vi "Test Driver.vi"() -> ()   [LabVIEW 2017]
uses:
  Controls/Test Driver States.ctl
  LabVIEW Library/Controls/Acquisition Modes.ctl
  LabVIEW Library/Controls/Acquisition Commands.ctl
  <vilib>/vision/Image Controls.llb/IMAQ Image.ctl
  builds/BonTechDetector.lvlibp
  LabVIEW Library/BonTechDetector.lvlib
  <vilib>/vision/NI_Vision_Development_Module.lvlib
panel:
  in  "byte order (0:big-endian, network order)":T1(ring)
  in  "Save Image":bool
  in  "Save File to":path
  out "SendCapCommand Status":i32 format="%.0x"
  in  "Acquisition Mode":T2(ring)
  in  "Stop Continuous Acquisition":bool
  in  "Start Continuous  Acquisition":bool
  in  "Acquisition Commands (nMode)":u16(ring) items=["ACQ_INIT"=0, "DARK_MODE"=1, "BRIGHT_MODE"=2, "SOFTTRIGGER_MODE"=258, "SOFTTRIGGER_INSTANT_MODE"=259]
  out "Continous Acq function Status":i32 format="%.0x"
  out "nHeight out":u32
  out "nWidth out":u32
  in  "Error in (no error)":errorcluster
  in  "Disconnect":bool
  in  "Capture Image":bool
  in  "Configure":bool
  in  "Connect":bool
  out "Capture Status":i32 format="%.0x"
  out "Image":T3(plugin-control)
  in  "CalRefPath":string="C:\\\\BSD\\\\192.168.3.240\\\\Reference"
  in  "ConfigDir":string="C:\\\\BSD\\\\192.168.3.240\\\\Config"
  out "lpszSerialNum out":string
  out "Acq Mode Set Status":i32 format="%.0x"
  out "Error out":errorcluster
  out "Disconnect Status":i32 format="%.0x"
  out "Connect Status":i32 format="%.0x"
  in  "nSensorIP":string="192.168.3.240"
  in  "nHostIP":string="192.168.3.5"
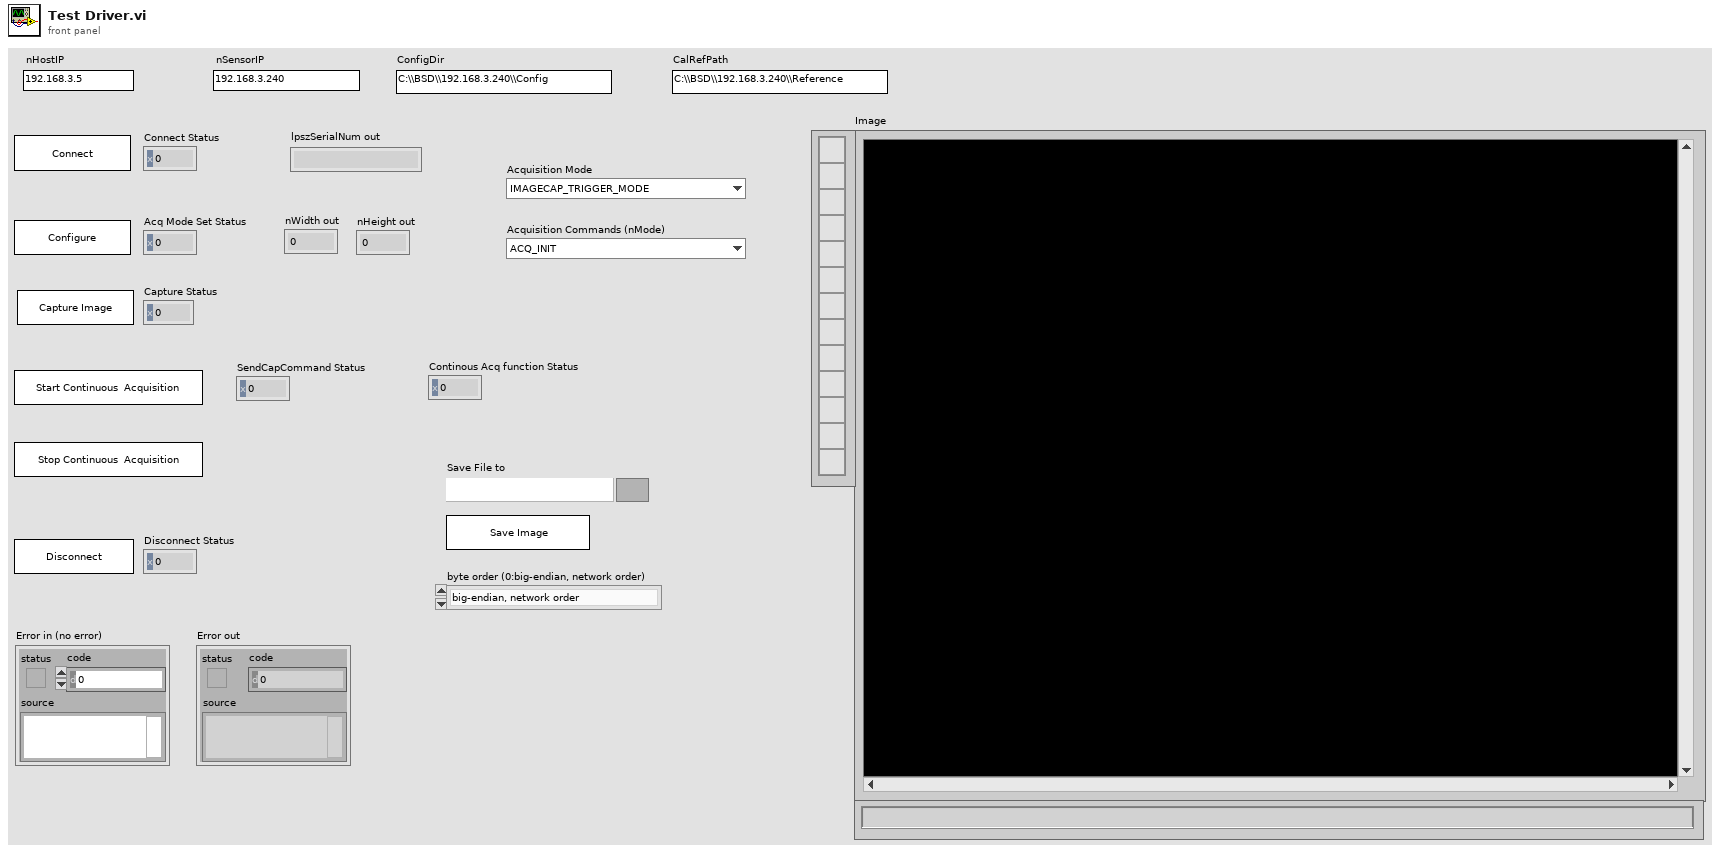
[diagram p1: front panel]
types:
  T1 = enum16{"big-endian, network order", "native, host order", "little-endian"}
  T2 = enum16{"IMAGECAP_TRIGGER_MODE", "IMAGECAP_AED_MODE", "IMAGECAP_SOFTTRIGGER_MODE", "IMAGECAP_AVG_COUNT_MODE", "IMAGECAP_AVG_AED_MODE", "IMAGECAP_CONTINUOUS_MODE", "IMAGECAP_CONTINUOUS_BINNING_MODE", "IMAGECAP_VIEWER_MODE"}
  T3 = typedef "IMAQ Image.ctl" = refnum<image>
  T4 = typedef "BonTechDetector.lvlib/Acquisition Modes.ctl" = enum32{"IMAGECAP_TRIGGER_MODE", "IMAGECAP_AED_MODE", "IMAGECAP_SOFTTRIGGER_MODE", "IMAGECAP_AVG_COUNT_MODE", "IMAGECAP_AVG_AED_MODE", "IMAGECAP_CONTINUOUS_MODE", "IMAGECAP_VIEWER_MODE", "IMAGECAP_CONTINUOUS_BINNING_MODE"}
  T5 = typedef "BonTechDetector.lvlib/Acquisition Commands.ctl" = u32
  T6 = cluster{"nHostIP String":string, "nSensorIP String":string, "ConfigDir":string, "CalRefPath":string, "nMode":T4, "nAcqCommand":T5, "pImage":u16[], "ImageRef":T3, "nWidth":u32, "nHeight":u32, "nHostIP":u32, "nSensorIP":u32, "imgCapQ":refnum<queue>}
  T7 = typedef "Test Driver States.ctl" = enum16{"Poll", "Init", "Connect", "Configure", "Capture Image", "Save Image", "Disconnect", "Error", "Exit"}
  T8 = typedef "Image Type" = u32
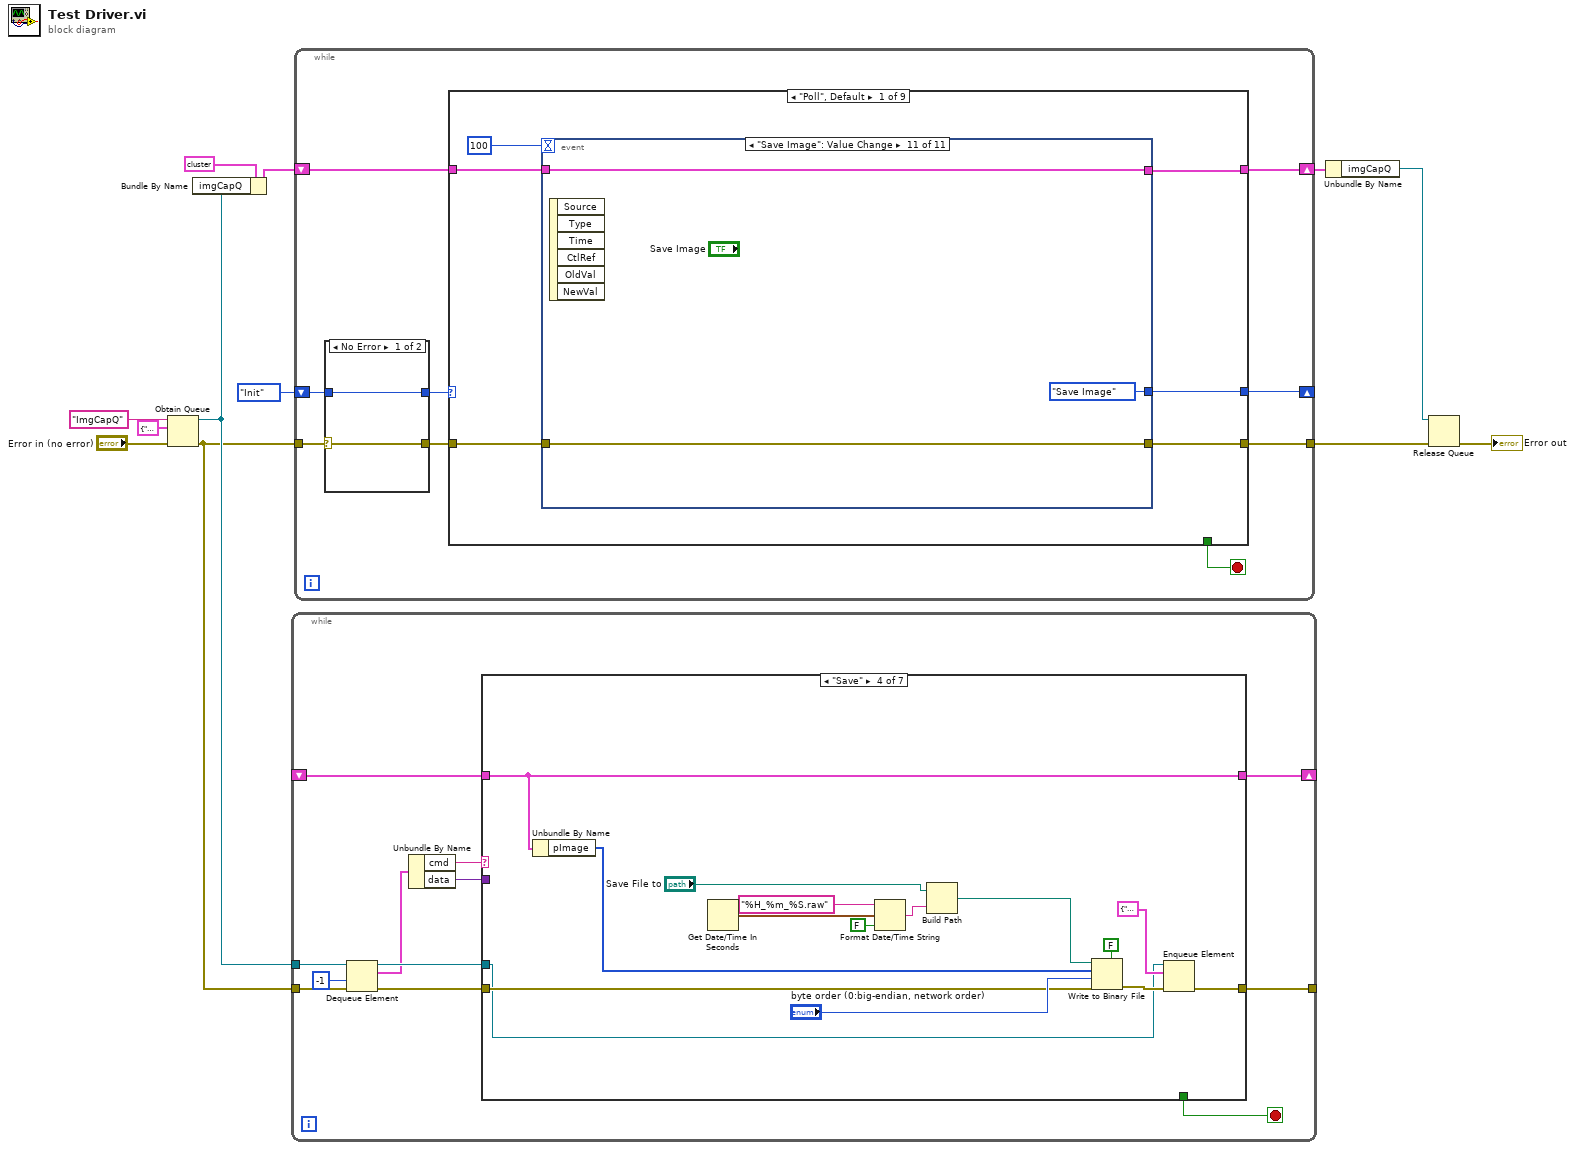
[diagram p0: block diagram]
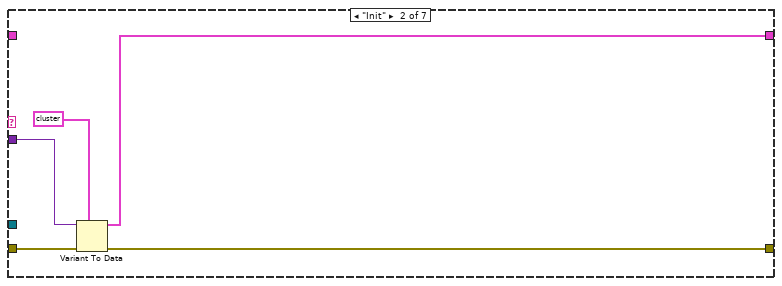
[diagram p3: hidden frame]
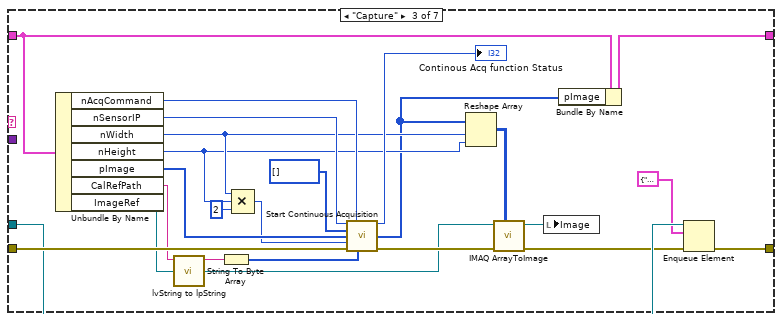
[diagram p4: hidden frame]
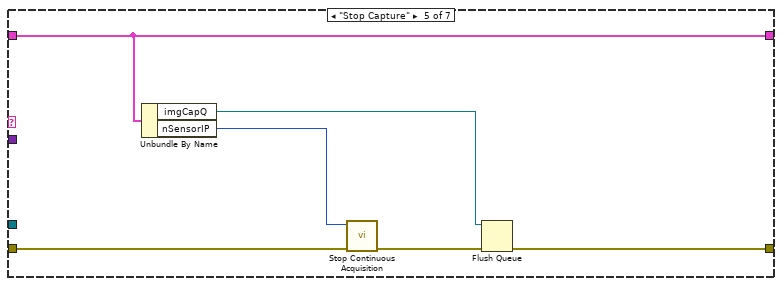
[diagram p5: hidden frame]
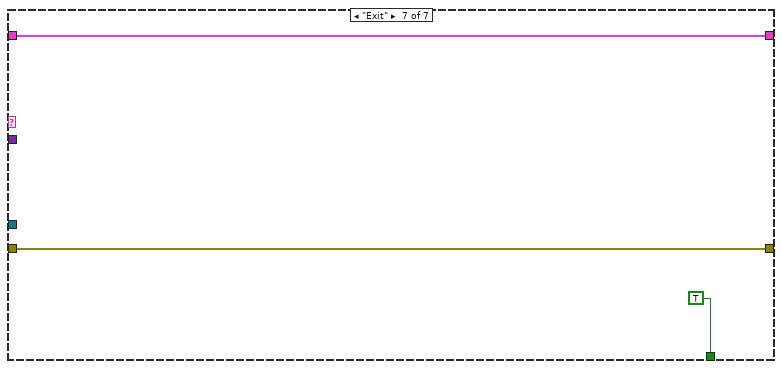
[diagram p7: hidden frame]
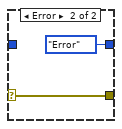
[diagram p8: hidden frame]
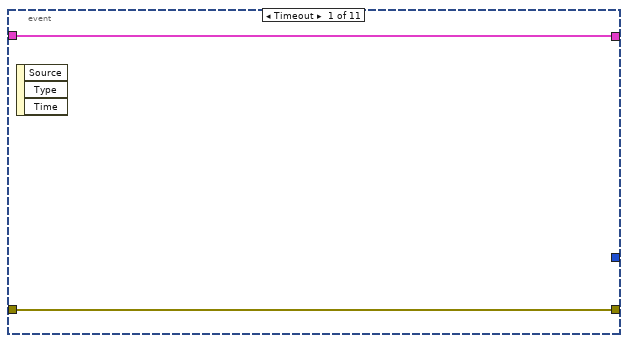
[diagram p9: hidden frame]
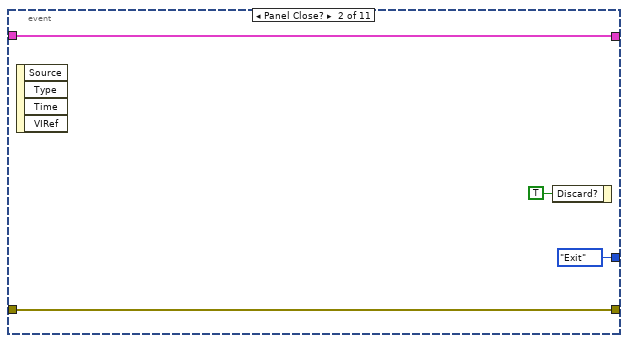
[diagram p10: hidden frame]
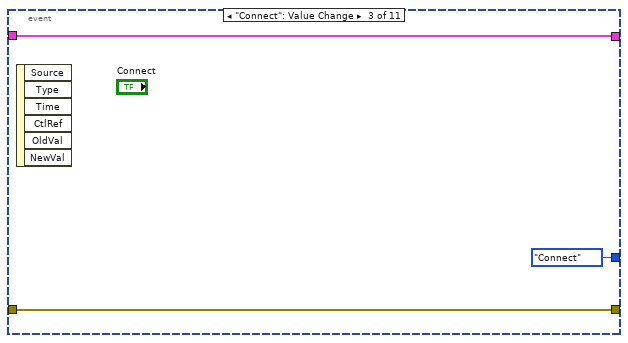
[diagram p11: hidden frame]
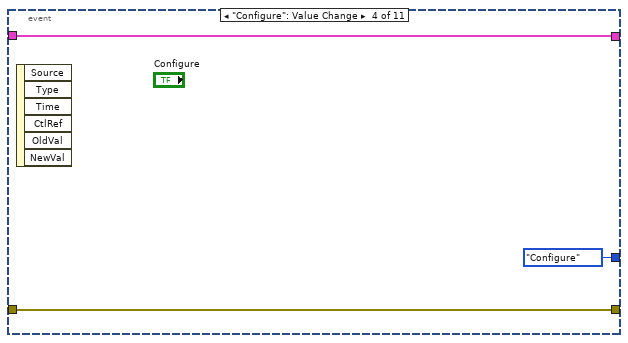
[diagram p12: hidden frame]
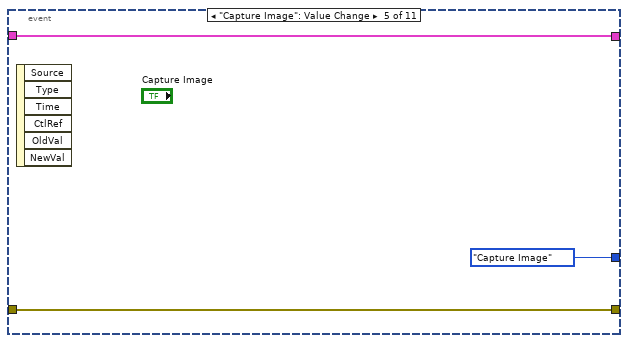
[diagram p13: hidden frame]
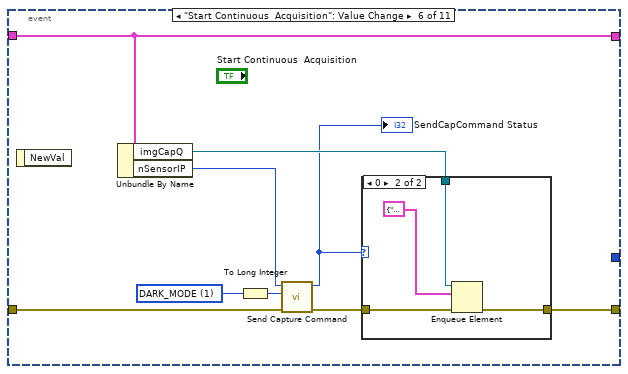
[diagram p14: hidden frame]
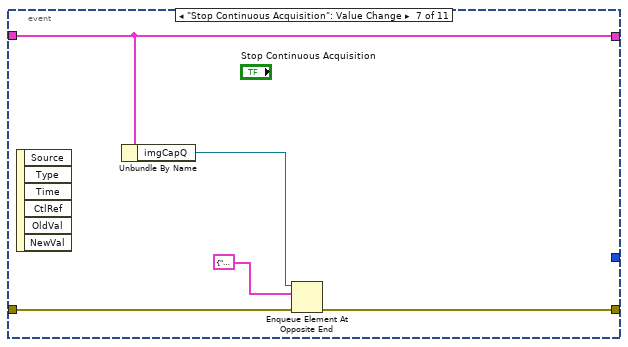
[diagram p16: hidden frame]
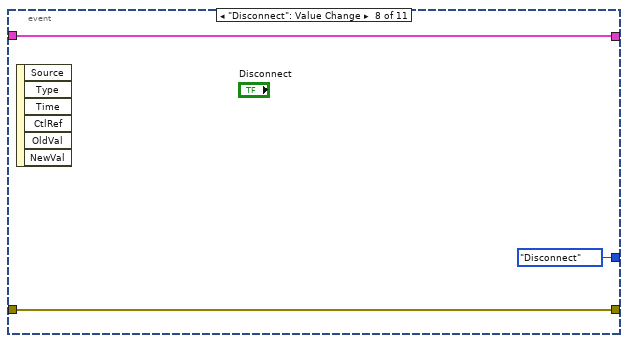
[diagram p17: hidden frame]
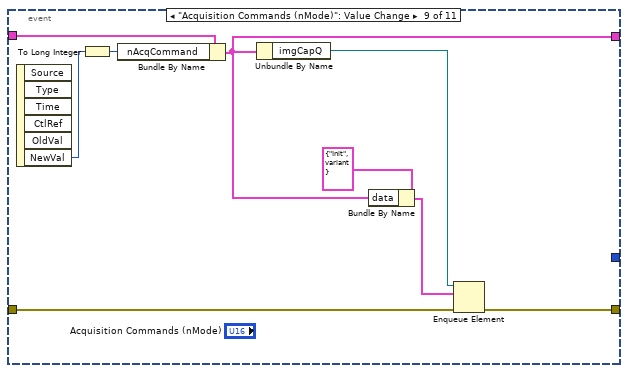
[diagram p18: hidden frame]
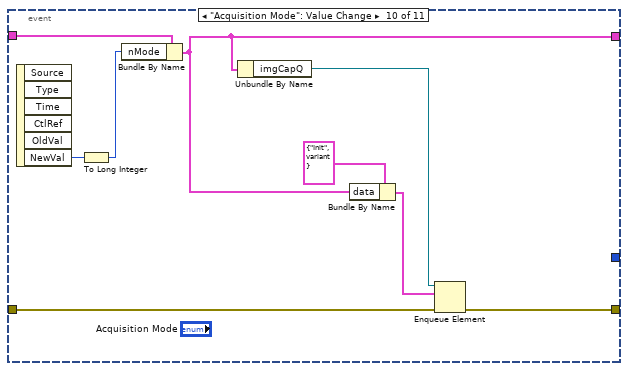
[diagram p19: hidden frame]
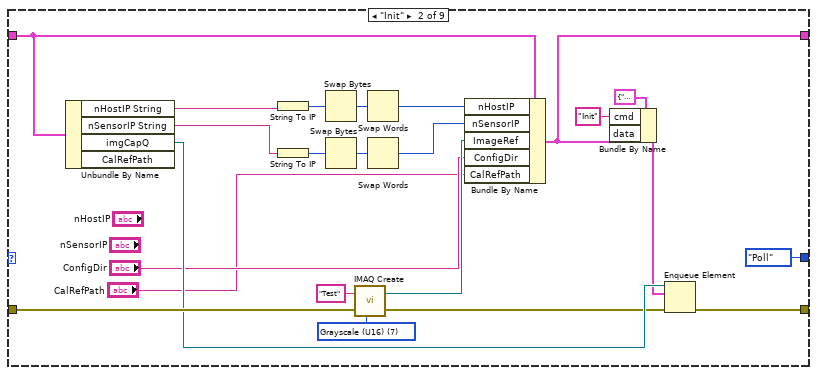
[diagram p20: hidden frame]
diagram:
  n1 = Obtain Queue(name (unnamed)="ImgCapQ", element data type=cluster{"cmd":string, "data":variant} {"cmd"="", "data"=variant}, error in (no error)="Error in (no error)") -> (queue out=w7:refnum<queue>, error out=w6:errorcluster)  [unwired: 2 in, 1 out]
  n2 = Bundle By Name(cluster=T6 {"nHostIP String"="192.168.3.5", "nSensorIP String"="192.168.3.240", "ConfigDir"="D:\\\\BSDx64\\\\192.168.3.240\\\\Config", "CalRefPath"="D:\\\\BSDx64\\\\192.168.3.240\\\\Reference", "nMode"=enum."IMAGECAP_CONTINUOUS_MODE", "nAcqCommand"=1, "pImage"=[], "ImageRef"=refnum, "nWidth"=3072, "nHeight"=3072, "nHostIP"=0, "nSensorIP"=0, "imgCapQ"=refnum}, "imgCapQ"=w7) -> (w8:T6)
  n3 = while {
    tunnel: w7 -> [w24]
    tunnel: w6 -> [w22]
    tunnel: [w19] -> _
    shift-right: [w14] -> _
    shift-left: _ -> [w13]
    stop <- w15 stop-if-true
    n4 = Dequeue Element(queue=w24, timeout in ms (-1)=-1, error in (no error)=w22) -> (queue out=w21:refnum<queue>, element=w18:cluster{"cmd":string, "data":variant}, error out=w20:errorcluster)  [unwired: 1 out]
    n5 = Unbundle By Name(w18) -> ("cmd"=w17:string, "data"=w16:variant)
    n6 = case shown="\"Save\"" w17 {
      tunnel: w21 -> [_ _ w45 w57 _ _ _]
      tunnel: w20 -> [w26 w31 w55 w67 w74 w77 w81]
      tunnel: [w26 w28 w43 w58 w71 w77 w81] -> w19
      tunnel: w16 -> [_ w30 _ _ _ _ _]
      tunnel: [_ _ _ _ _ _ TRUE] -> w15
      tunnel: [w25 w29 w33 w70 w76 w78 w79] -> w14
      tunnel: w13 -> [w25 _ w54 w70 w76 w78 w79]
      frame "Idle", Default {
      }
      frame "Init" {
        n7 = Variant To Data(error in=w31, type=T6 {"nHostIP String"="192.168.3.5", "nSensorIP String"="192.168.3.240", "ConfigDir"="D:\\\\BSDx64\\\\192.168.3.240\\\\Config", "CalRefPath"="D:\\\\BSDx64\\\\192.168.3.240\\\\Reference", "nMode"=enum."IMAGECAP_CONTINUOUS_MODE", "nAcqCommand"=1, "pImage"=[], "ImageRef"=refnum, "nWidth"=3072, "nHeight"=3072, "nHostIP"=0, "nSensorIP"=0, "imgCapQ"=refnum}, Variant=w30) -> (data=w29:T6, error out=w28:errorcluster)
      }
      frame "Capture" {
        n8 = Unbundle By Name(w54) -> ("nAcqCommand"=w41:T5, "nSensorIP"=w53:u32, "nWidth"=w37:u32, "nHeight"=w36:u32, "pImage"=w51:u16[], "CalRefPath"=w35:string, "ImageRef"=w46:T3)
        n9 = call "lvString to lpString.vi"("LVString"=w35) -> ("LPTSTR String"=w34:string)  [unwired: 10 in]
        n10 = String To Byte Array(string=w34) -> (unsigned byte array=w40:u8[])
        n11 = Compound Arithmetic op=MULTIPLY(w37, w36, u32 2 ("value")) -> (w38:u32)
        n12 = call "Start Continuous Acquisition.vi"("nSensorIP"=w53, "nMode"=w41, "refImg"=u16[] [], "pImg"=w51, "nBuffLength"=w38, "error in (no error)"=w55, "lpszRefPath"=w40) -> ("function return"=→"Continous Acq function Status":i32, "pImg out"=w32:u16[], "error out"=w50:errorcluster)  [unwired: 5 in, 1 out]
        n13 = Reshape Array(w32, w37, w36) -> (w49:u16[][])
        n14 = call "IMAQ ArrayToImage"("Image Pixels (U16)"=w49, "error in (no error)"=w50, "Image"=w46) -> ("error out"=w44:errorcluster, "Image Out"=w47:T3)  [unwired: 7 in]
        n15 = local write "Image"(w47) -> ()
        n16 = Bundle By Name(cluster=w54, "pImage"=w32) -> (w33:T6)
        n17 = Enqueue Element(queue=w45, element=cluster{"cmd":string, "data":variant} {"cmd"="Capture", "data"=variant}, error in (no error)=w44) -> (error out=w43:errorcluster)  [unwired: 1 in, 2 out]
      }
      frame "Save" {
        n18 = Unbundle By Name(w70) -> ("pImage"=w69:u16[])
        n19 = Get Date/Time In Seconds() -> (seconds since 1Jan1904=w66:timestamp)
        n20 = Format Date/Time String(time format string (%c)="%H_%m_%S.raw", seconds (now)=w66, UTC format=FALSE) -> (date/time string=w63:string)
        n21 = Build Path(base path="Save File to", name or relative path=w63) -> (appended path=w61:path)
        n22 = Write to Binary File(file (use dialog)=w61, data=w69, error in=w67, 5:FALSE ("prepend array or string size? (T)"), 9:"byte order (0:big-endian, network order)") -> (error out=w59:errorcluster)  [unwired: 1 in, 2 out]
        n23 = Enqueue Element(queue=w57, element=cluster{"cmd":string, "data":variant} {"cmd"="Capture", "data"=variant}, error in (no error)=w59) -> (error out=w58:errorcluster)  [unwired: 1 in, 2 out]
      }
      frame "Stop Capture" {
        n24 = Unbundle By Name(w76) -> ("imgCapQ"=w73:refnum<queue>, "nSensorIP"=w75:u32)
        n25 = call "Stop Continuous Acquisition.vi"("error in (no error)"=w74, "nSensorIP"=w75) -> ("error out"=w72:errorcluster)  [unwired: 8 in, 1 out]
        n26 = Flush Queue(queue=w73, error in (no error)=w72) -> (error out=w71:errorcluster)  [unwired: 2 out]
      }
      frame "Error" {
      }
      frame "Exit" {
      }
    }
  }
  n27 = while {
    shift-right: [w82] -> _
    shift-left: Test_Driver_States."Init" -> [w86]
    tunnel: w6 -> [w90]
    shift-right: [w88] -> w3
    shift-left: w8 -> [w89]
    tunnel: [w84] -> w5
    stop <- w83 stop-if-true
    n28 = case shown="No Error" w90 {
      selector: w90 -> [w92 w94]
      tunnel: [w92 w94] -> w87
      tunnel: w86 -> [w91 _]
      tunnel: [w91 Test_Driver_States."Error"] -> w85
      frame No Error {
      }
      frame Error {
      }
    }
    n29 = case shown="\"Poll\", Default" w85 {
      tunnel: w89 -> [w99 w178 w199 w228 w231 w236 w248 w258 w261]
      tunnel: [w98 w162 w182 w223 w231 w236 w248 w258 w261] -> w88
      tunnel: w87 -> [w97 w179 w200 w229 w230 w237 w250 w254 w262]
      tunnel: [w96 w164 w184 w210 w230 w234 w249 w255 w259] -> w84
      tunnel: [_ _ _ _ _ TRUE _ _ _] -> w83
      tunnel: [w95 Test_Driver_States."Poll" _ _ _ _ _ Test_Driver_States."Poll" _] -> w82
      frame "Poll", Default {
        n30 = event shown="[10] \"Save Image\": Value Change" {
          selector: _ -> [_ _ _ _ _ _ _ _ _ _ _]
          dyn-events: _ -> [_ _ _ _ _ _ _ _ _ _ _]
          timeout: 100 -> [_ _ _ _ _ _ _ _ _ _ _]
          tunnel: [w102 w106 w109 w111 w115 w123 w132 w137 w139 w147 w158] -> w98
          tunnel: w99 -> [w102 w106 w109 w111 w115 w123 w132 w137 w146 w148 w158]
          tunnel: w97 -> [w101 w103 w107 w112 w114 w124 w134 w136 w142 w150 w157]
          tunnel: [w101 w103 w107 w112 w114 w118 w133 w136 w141 w149 w157] -> w96
          tunnel: [_ Test_Driver_States."Exit" Test_Driver_States."Connect" Test_Driver_States."Configure" Test_Driver_States."Capture Image" _ _ Test_Driver_States."Disconnect" _ _ Test_Driver_States."Save Image"] -> w95
          event Timeout {
            n31 = event-data() -> ()  [unwired: 1 in, 3 out]
          }
          event Panel Close? {
            n32 = event-data() -> ()  [unwired: 1 in, 4 out]
            n33 = event-data("Discard?"=TRUE) -> ()  [unwired: 1 in, 1 out]
          }
          event "Connect": Value Change {
            n34 = event-data() -> ()  [unwired: 1 in, 6 out]
          }
          event "Configure": Value Change {
            n35 = event-data() -> ()  [unwired: 1 in, 6 out]
          }
          event "Capture Image": Value Change {
            n36 = event-data() -> ()  [unwired: 1 in, 6 out]
          }
          event "Start Continuous  Acquisition": Value Change {
            w121 = u16 1 items=["ACQ_INIT"=0, "DARK_MODE"=1, "BRIGHT_MODE"=2, "SOFTTRIGGER_MODE"=258, "SOFTTRIGGER_INSTANT_MODE"=259] ("Acquisition Commands (nMode)")
            n37 = event-data() -> ()  [unwired: 1 in, 1 out]
            n38 = Unbundle By Name(w123) -> ("imgCapQ"=w117:refnum<queue>, "nSensorIP"=w122:u32)
            n39 = To Long Integer(number=w121) -> (32bit integer=w120:i32)
            n40 = call "Send Capture Command.vi"("error in (no error)"=w124, "nCmd"=w120, "nSensorIP"=w122) -> ("error out"=w119:errorcluster, "function return"=w116:i32)  [unwired: 7 in]
            "SendCapCommand Status" <- w116
            n41 = case shown="0" w116 {
              tunnel: w119 -> [w125 w129]
              tunnel: [w125 w128] -> w118
              tunnel: w117 -> [_ w127]
              frame 1, Default {
              }
              frame 0 {
                n42 = Enqueue Element(queue=w127, element=cluster{"cmd":string, "data":variant} {"cmd"="Capture", "data"=variant}, error in (no error)=w129) -> (error out=w128:errorcluster)  [unwired: 1 in, 2 out]
              }
            }
          }
          event "Stop Continuous Acquisition": Value Change {
            n43 = event-data() -> ()  [unwired: 1 in, 6 out]
            n44 = Unbundle By Name(w132) -> ("imgCapQ"=w131:refnum<queue>)
            n45 = Enqueue Element At Opposite End(queue=w131, element=cluster{"cmd":string, "data":variant} {"cmd"="Stop Capture", "data"=variant}, error in (no error)=w134) -> (error out=w133:errorcluster)  [unwired: 1 in, 2 out]
          }
          event "Disconnect": Value Change {
            n46 = event-data() -> ()  [unwired: 1 in, 6 out]
          }
          event "Acquisition Commands (nMode)": Value Change {
            n47 = event-data() -> ("NewVal"=w145:u16)  [unwired: 1 in, 5 out]
            n48 = To Long Integer(number=w145) -> (32bit integer=w144:i32)
            n49 = Bundle By Name(cluster=w146, "nAcqCommand"=w144) -> (w139:T6)
            n50 = Unbundle By Name(w139) -> ("imgCapQ"=w138:refnum<queue>)
            n51 = Bundle By Name(cluster=cluster{"cmd":string, "data":variant} {"cmd"="Init", "data"=variant} ("element"), "data"=w139) -> (w140:cluster{"cmd":string, "data":variant})
            n52 = Enqueue Element(queue=w138, element=w140, error in (no error)=w142) -> (error out=w141:errorcluster)  [unwired: 1 in, 2 out]
          }
          event "Acquisition Mode": Value Change {
            n53 = event-data() -> ("NewVal"=w155:T2)  [unwired: 1 in, 5 out]
            n54 = To Long Integer(number=w155) -> (32bit integer=w154:i32)
            n55 = Bundle By Name(cluster=w148, "nMode"=w154) -> (w147:T6)
            n56 = Unbundle By Name(w147) -> ("imgCapQ"=w152:refnum<queue>)
            n57 = Bundle By Name(cluster=cluster{"cmd":string, "data":variant} {"cmd"="Init", "data"=variant} ("element"), "data"=w147) -> (w153:cluster{"cmd":string, "data":variant})
            n58 = Enqueue Element(queue=w152, element=w153, error in (no error)=w150) -> (error out=w149:errorcluster)  [unwired: 1 in, 2 out]
          }
          event "Save Image": Value Change {
            n59 = event-data() -> ()  [unwired: 1 in, 6 out]
          }
        }
      }
      frame "Init" {
        w180 = T8 7 items=["Grayscale (U8)", "Grayscale (I16)", "Grayscale (SGL)", "Complex (CSG)", "RGB (U32)", "HSL (U32)", "RGB (U64)", "Grayscale (U16)"] ("Image Type")
        n60 = Unbundle By Name(w178) -> ("nHostIP String"=w173:string, "nSensorIP String"=w172:string, "imgCapQ"=w167:refnum<queue>)  [unwired: 1 out]
        n61 = String To IP(1:w173) -> (0:w176:u32)
        n62 = String To IP(1:w172) -> (0:w177:u32)
        n63 = Swap Bytes(anything=w176) -> (byte swapped=w175:u32)
        n64 = Swap Bytes(anything=w177) -> (byte swapped=w174:u32)
        n65 = call "IMAQ Create"("Image Name"="Test", "Image Type"=w180, "error in (no error)"=w179) -> ("New Image"=w169:T3, "error out"=w165:errorcluster)  [unwired: 2 in]
        n66 = Swap Words(1:w175) -> (0:w170:u32)
        n67 = Swap Words(1:w174) -> (0:w171:u32)
        n68 = Bundle By Name(cluster=w178, "nHostIP"=w170, "nSensorIP"=w171, "ImageRef"=w169, "ConfigDir"="ConfigDir", "CalRefPath"="CalRefPath") -> (w162:T6)
        n69 = Bundle By Name(cluster=cluster{"cmd":string, "data":variant} {"cmd"="", "data"=variant} ("element"), "cmd"="Init", "data"=w162) -> (w163:cluster{"cmd":string, "data":variant})
        n70 = Enqueue Element(queue=w167, element=w163, error in (no error)=w165) -> (error out=w164:errorcluster)  [unwired: 1 in, 2 out]
      }
      frame "Configure" {
        n71 = Unbundle By Name(w199) -> ("nSensorIP"=w198:u32, "nMode"=w194:T4, "imgCapQ"=w183:refnum<queue>)
        n72 = disable-structure shown="Enabled" {
          disable-tunnel: [w208 w209] -> w203
          disable-tunnel: w200 -> [w207 w209]
          disable-tunnel: w198 -> [w206 _]
          disable-tunnel: [w205 _] -> w195
          disable-tunnel: w194 -> [w204 _]
          frame Enabled {
            n73 = call "Set Acquisition Mode.vi"("error in (no error)"=w207, "nMode"=w204, "nSensorIP"=w206) -> ("error out"=w208:errorcluster, "function return"=w205:i32)  [unwired: 7 in]
          }
          frame Disabled {
          }
        }
        "Acq Mode Set Status" <- w195
        n74 = call "Get Frame Size.vi"("error in (no error)"=w203, "nHeight"=u16 0, "nWidth"=u16 0, "nSensorIP"=w198) -> ("error out"=w185:errorcluster, "nHeight out"=w196:u16, "nWidth out"=w197:u16)  [unwired: 4 in, 1 out]
        n75 = To Unsigned Long Integer(number=w197) -> (unsigned 32bit integer=w190:u32)
        "nWidth out" <- w190
        n76 = To Unsigned Long Integer(number=w196) -> (unsigned 32bit integer=w193:u32)
        "nHeight out" <- w193
        n77 = Multiply(x=w190, y=w190) -> (x*y=w189:u32)
        n78 = Initialize Array(u16 0 ("element"), w189) -> (w192:u16[])
        n79 = Bundle By Name(cluster=w199, "nWidth"=w190, "nHeight"=w193, "pImage"=w192) -> (w182:T6)
        n80 = Bundle By Name(cluster=cluster{"cmd":string, "data":variant} {"cmd"="", "data"=variant} ("element"), "cmd"="Init", "data"=w182) -> (w188:cluster{"cmd":string, "data":variant})
        n81 = Enqueue Element(queue=w183, element=w188, error in (no error)=w185) -> (error out=w184:errorcluster)  [unwired: 1 in, 2 out]
      }
      frame "Capture Image" {
        n82 = Unbundle By Name(w228) -> ("CalRefPath"=w226:string, "nSensorIP"=w227:u32, "pImage"=w224:u16[], "ImageRef"=w219:T3, "nAcqCommand"=w217:T5, "nWidth"=w215:u32, "nHeight"=w214:u32)
        n83 = call "lvString to lpString.vi"("LVString"=w226) -> ("LPTSTR String"=w225:string)  [unwired: 10 in]
        n84 = String To Byte Array(string=w225) -> (unsigned byte array=w216:u8[])
        n85 = call "Capture Single Image.vi"("calRefPath"=w216, "nMode"=w217, "nWidth"=w215, "error in (no error)"=w229, "nHeight"=w214, "pImage"=w224, "nSensorIP"=w227) -> ("error out"=w220:errorcluster, "pImage out"=w221:u16[], "function return"=→"Capture Status":i32)  [unwired: 2 in]
        n86 = Bundle By Name(cluster=w228, "pImage"=w221) -> (w223:T6)
        n87 = Reshape Array(w221, w215, w214) -> (w222:u16[][])
        n88 = call "IMAQ ArrayToImage"("Image Pixels (U16)"=w222, "error in (no error)"=w220, "Image"=w219) -> ("error out"=w212:errorcluster, "Image Out"=w213:T3)  [unwired: 7 in]
        n89 = call "IMAQ Inverse"("error in (no error)"=w212, "Image Src"=w213) -> ("error out"=w210:errorcluster, "Image Dst Out"=→"Image":T3)  [unwired: 8 in]
      }
      frame "Error" {
      }
      frame "Exit" {
        n90 = Unbundle By Name(w236) -> ("imgCapQ"=w233:refnum<queue>, "ImageRef"=w235:T3)
        n91 = call "IMAQ Dispose"("Image"=w235, "error in (no error)"=w237) -> ("error out"=w234:errorcluster)  [unwired: 4 in]
        n92 = invoke class="VI" method="Default Vals.Reinit All"() -> ()  [unwired: 3 in, 3 out]
        n93 = Enqueue Element(queue=w233, element=cluster{"cmd":string, "data":variant} {"cmd"="Exit", "data"=variant}) -> ()  [unwired: 2 in, 3 out]
      }
      frame "Connect" {
        n94 = Unbundle By Name(w248) -> ("nHostIP"=w247:u32, "nSensorIP"=w244:u32, "ConfigDir"=w246:string)
        n95 = call "lvString to lpString.vi"("LVString"=w246) -> ("LPTSTR String"=w245:string)  [unwired: 10 in]
        n96 = String To Byte Array(string=w245) -> (unsigned byte array=w241:u8[])
        n97 = call "Connect.vi"("error in (no error)"=w250, "ConfigDir"=w241, "nSensorIP"=w244, "nHostIP"=w247) -> ("error out"=w251:errorcluster, "function return"=→"Connect Status":i32)  [unwired: 6 in]
        n98 = call "Get Serial Number.vi"("error in (no error)"=w251, "nSensorIP"=w244) -> ("error out"=w249:errorcluster, "lpszSerialNum out"=w242:u8[])  [unwired: 7 in, 1 out]
        n99 = Byte Array To String(unsigned byte array=w242) -> (string=w240:string)
        n100 = call "lpString to lvString.vi"("LPTSTR String"=w240) -> ("LVString"=→"lpszSerialNum out":string)  [unwired: 10 in]
      }
      frame "Disconnect" {
        n101 = Unbundle By Name(w258) -> ("nSensorIP"=w252:u32)
        n102 = call "Capture Single Image.vi"("error in (no error)"=w254, "nSensorIP"=w252) -> ("error out"=w253:errorcluster)  [unwired: 7 in, 2 out]
        n103 = call "Disconnect.vi"("error in (no error)"=w253, "nSensorIP"=w252) -> ("error out"=w255:errorcluster, "function return"=→"Disconnect Status":i32)  [unwired: 8 in]
        n104 = invoke class="VI" method="Default Vals.Reinit All"(error in=w255) -> ()  [unwired: 2 in, 3 out]
      }
      frame "Save Image" {
        n105 = Unbundle By Name(w261) -> ("imgCapQ"=w260:refnum<queue>)
        n106 = Enqueue Element(queue=w260, element=cluster{"cmd":string, "data":variant} {"cmd"="Save", "data"=variant}, error in (no error)=w262) -> (error out=w259:errorcluster)  [unwired: 1 in, 2 out]
      }
    }
  }
  n107 = Unbundle By Name(w3) -> ("imgCapQ"=w2:refnum<queue>)
  n108 = Release Queue(queue=w2, error in (no error)=w5) -> (error out=→"Error out":errorcluster)  [unwired: 1 in, 2 out]
